vi "Prompt for Step.vi"(8 "error in (no error)":errorcluster, 9 "Exit Event":refnum<user-event>, 10 "Subpanel Ref":refnum<vi>, 11 "Window Action in":refnum<class "Window Action.lvclass">) -> (0 "error out":errorcluster, 2 "OK?":bool, 3 "Window Action out":refnum<class "Window Action.lvclass">)   [LabVIEW 2020, in "MacroAssert.lvlib" / "Window Action.lvclass"]
uses:
  Window Action.lvclass
  Window Action.lvclass/Window Action.ctl
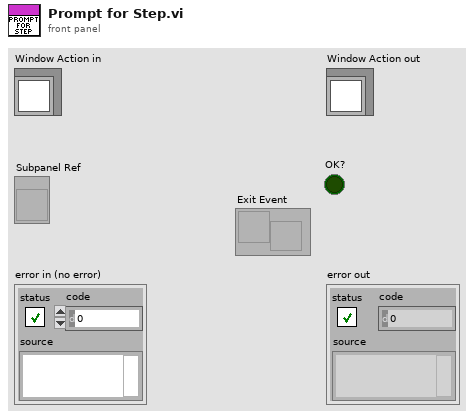
[diagram p1: front panel]
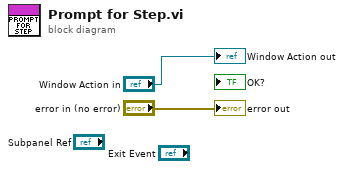
[diagram p0: block diagram]
diagram:
  "error out" <- "error in (no error)"
  "Window Action out" <- "Window Action in"
